vi "Corners to Rectangle.vi"(10 "tag info":T1={"tag ID"=0, "Center"={"X"=0.0, "Y"=0.0}, "homography matrix"=[], "decision margin"=0.0, "Hamming Dist"=0, "corner points"=[], "Tag Family"="36h11"}) -> (2 "output cluster":T2={"diameter points"={"first point"={"x"=0.0, "y"=0.0}, "projected point"={"x"=0.0, "y"=0.0}}, "normalized center"={"x"=0.0, "y"=0.0}, "Overall Score"=0.0, "Distance (in)"=0.0, "Offset Angle"=0.0, "Tag corner points"=[], "Tag Center"={"X"=0.0, "Y"=0.0}, "Tag Yaw"=0.0, "Tag Pitch"=0.0, "Target Roll (deg)"=0.0, "AprilTag Number"=68, "homography matrix"=[]} {"Tag Center"."Y" format="%0.2f"; "Tag Center"."X" format="%0.2f"})   [LabVIEW 2025]
uses:
  AprilTag Target Fields.ctl
panel:
  # "Bottom Left"
  # "Bottom Right"
  # "Top Right"
  # "Top Left"
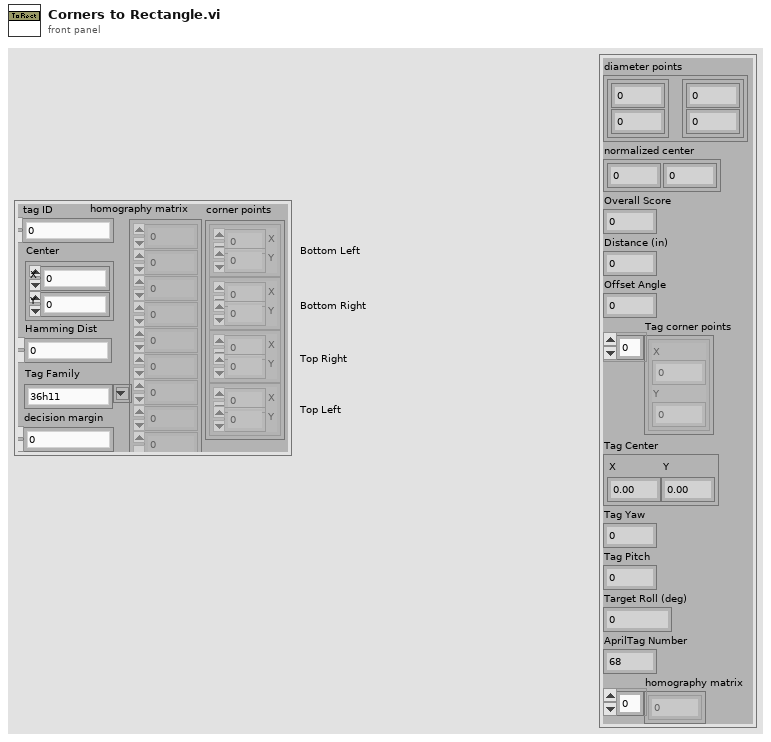
[diagram p1: front panel]
types:
  T1 = cluster{"tag ID":i32, "Center":cluster{"X":dbl, "Y":dbl}, "homography matrix":dbl[], "decision margin":dbl, "Hamming Dist":i32, "corner points":cluster{"X":dbl, "Y":dbl}[], "Tag Family":string}
  T2 = typedef "AprilTag Target Fields.ctl" = cluster{"diameter points":cluster{"first point":cluster{"x":dbl, "y":dbl}, "projected point":cluster{"x":dbl, "y":dbl}}, "normalized center":cluster{"x":dbl, "y":dbl}, "Overall Score":dbl, "Distance (in)":dbl, "Offset Angle":dbl, "Tag corner points":cluster{"X":dbl, "Y":dbl}[], "Tag Center":cluster{"X":dbl, "Y":dbl}, "Tag Yaw":dbl, "Tag Pitch":dbl, "Target Roll (deg)":dbl, "AprilTag Number":i32, "homography matrix":dbl[]}
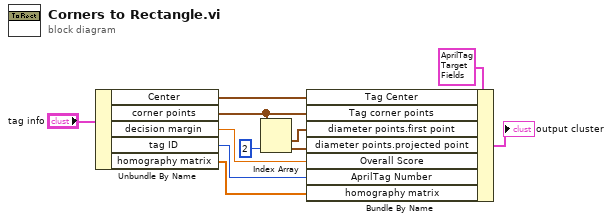
[diagram p0: block diagram]
diagram:
  n1 = Unbundle By Name("tag info") -> ("Center"=w4:cluster{"X":dbl, "Y":dbl}, "corner points"=w3:cluster{"X":dbl, "Y":dbl}[], "decision margin"=w5:dbl, "tag ID"=w2:i32, "homography matrix"=w1:dbl[])
  n2 = Index Array(array=w3, index #2=2 ("index")) -> (element #1=w10:cluster{"X":dbl, "Y":dbl}, element #2=w9:cluster{"X":dbl, "Y":dbl})  [unwired: 1 in]
  n3 = Bundle By Name(cluster=T2 {"diameter points"={"first point"={"x"=0.0, "y"=0.0}, "projected point"={"x"=0.0, "y"=0.0}}, "normalized center"={"x"=0.0, "y"=0.0}, "Overall Score"=0.0, "Distance (in)"=0.0, "Offset Angle"=0.0, "Tag corner points"=[], "Tag Center"={"X"=0.0, "Y"=0.0}, "Tag Yaw"=0.0, "Tag Pitch"=0.0, "Target Roll (deg)"=0.0, "AprilTag Number"=68, "homography matrix"=[]} ("results"), "Tag Center"=w4, "Tag corner points"=w3, "diameter points.first point"=w10, "diameter points.projected point"=w9, "Overall Score"=w5, "AprilTag Number"=w2, "homography matrix"=w1) -> (→"output cluster":T2)
